vi "Get Next Point.vi"(0 "eye scan point iterator":refnum<class "niHighSpeedSerial Rectangular Eye Scan Point Iterator v1 Host.lvclass">, 11 "error in":errorcluster) -> (4 "eye scan point iterator out":refnum<class "niHighSpeedSerial Rectangular Eye Scan Point Iterator v1 Host.lvclass">, 6 "next point":T1, 15 "error out":errorcluster)   [LabVIEW 2014, in "niHighSpeedSerial Rectangular Eye Scan Point Iterator v1 Host.lvclass"]
doc: "Advances to the next point to be measured and returns its horizontal and vertical offset.\n\n<B>Input Parameters</B>\n\n<B>eye scan point iterator</B> is the incoming wire for the Eye Scan Point Iterator class object\n\n<B>error in</B> describes error conditions that occur before this node runs. This input provides standard 'error in' functionality.\n\n<B>Output Parameters</B>\n\n<B>eye scan point iterator out</B> is the outgoing wire for the Eye Scan Point Iterator class object\n\n<B>next point</B> is the next point to being measuring using Eye Scan\n\n<B>next point.horizontal offset</B> is the horizontal offset of the next point.\n\n<B>next point.vertical offset</B> is the vertical offset of the next point.\n\n<B>error out</B> contains error information. This output provides standard 'error out' functionality."
uses:
  <instrlib>/niHighSpeedSerial/Eye Scan/v1/Host/Impl/Rect Iter/niHighSpeedSerial Rectangular Eye Scan Point Iterator v1 Host.lvclass
  <instrlib>/niHighSpeedSerial/Eye Scan/v1/Host/Common/Public/Point Offsets.ctl
  <instrlib>/niHighSpeedSerial/Eye Scan/v1/Host/Impl/Rect Iter/niHighSpeedSerial Rectangular Eye Scan Point Iterator v1 Host.lvclass/niHighSpeedSerial Rectangular Eye Scan Point Iterator v1 Host.ctl
  <instrlib>/niHighSpeedSerial/Eye Scan/v1/Host/Common/niHighSpeedSerial Eye Scan Common v1 Host.lvlib
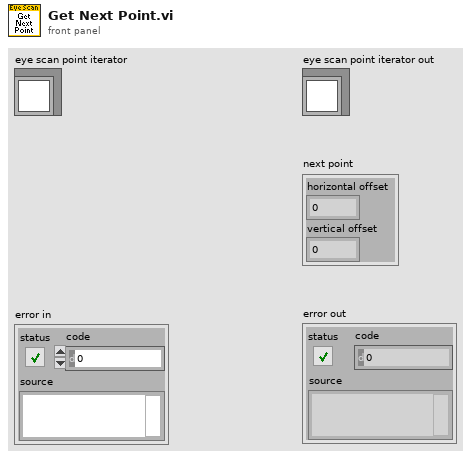
[diagram p1: front panel]
types:
  T1 = typedef "niHighSpeedSerial Eye Scan Common v1 Host.lvlib/Point Offsets.ctl" = cluster{"horizontal offset":i16, "vertical offset":i8}
  T2 = typedef "niHighSpeedSerial Eye Scan Common v1 Host.lvlib/Point.ctl" = cluster{"point offsets":T1, "sample count":u64, "error count":u64, "bit error rate":dbl}
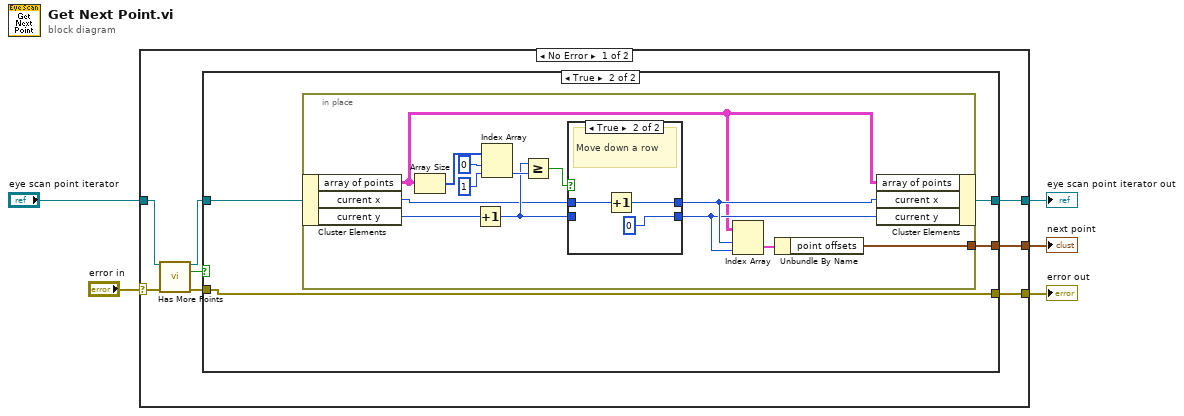
[diagram p0: block diagram]
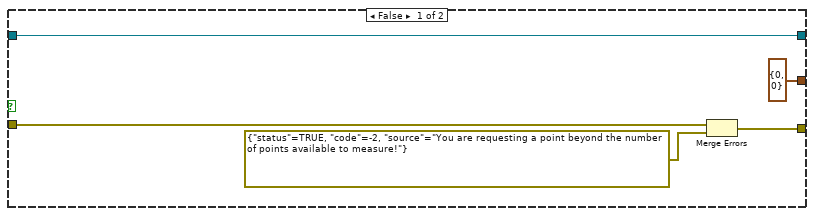
[diagram p2: hidden frame]
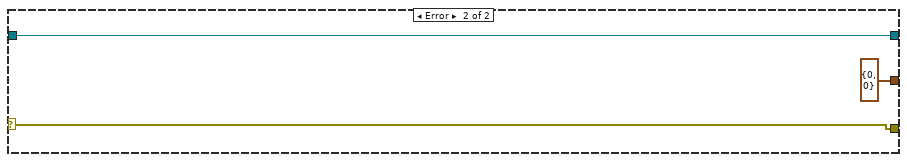
[diagram p4: hidden frame]
diagram:
  n1 = case shown="No Error" "error in" {
    selector: "error in" -> [w8 w43]
    tunnel: [w12 w43] -> w4
    tunnel: [w13 w42] -> w3
    tunnel: "eye scan point iterator" -> [w11 w42]
    tunnel: [w6 T1 {"horizontal offset"=0, "vertical offset"=0} ("Next Point")] -> w1
    frame No Error {
      n2 = call-dynamic "Has More Points.vi"("eye scan point iterator"=w11, "error in"=w8) -> ("eye scan point iterator out"=w10:refnum<class "niHighSpeedSerial Rectangular Eye Scan Point Iterator v1 Host.lvclass">, "has more points?"=w9:bool, "error out"=w7:errorcluster)  [unwired: 11 in]
      n3 = case shown="True" w9 {
        tunnel: [w15 w19] -> w13
        tunnel: [w16 w22] -> w12
        tunnel: w7 -> [w18 w22]
        tunnel: w10 -> [w15 w21]
        tunnel: [T1 {"horizontal offset"=0, "vertical offset"=0} ("Point Offsets") w20] -> w6
        frame False {
          n4 = Merge Errors(w18, errorcluster {"status"=TRUE, "code"=-2, "source"="You are requesting a point beyond the number of points available to measure!"} ("error out")) -> (w16:errorcluster)
        }
        frame True {
          n5 = in-place {
            in-place-border: [w23] -> w20
            n6 = in-place-cluster #1(w21) -> ("array of points"=w24:T2[][], "current x"=w28:i32, "current y"=w27:i32)
            n7 = Array Size(array=w24) -> (size(s)=w30:i32[])
            n8 = Increment(x=w27) -> (x+1=w34:i32)
            n9 = Index Array(array=w30, index #1=0 ("index"), index #2=1 ("index")) -> (element #2=w35:i32)  [unwired: 1 out]
            n10 = Greater Or Equal?(x=w34, y=w35) -> (x >= y?=w33:bool)
            n11 = case shown="True" w33 {
              tunnel: w28 -> [w36 w39]
              tunnel: [w37 0] -> w25
              tunnel: w34 -> [w37 _]
              tunnel: [w36 w38] -> w26
              frame False {
                # "Advance along the row"
              }
              frame True {
                # "Move down a row"
                n12 = Increment(x=w39) -> (x+1=w38:i32)
              }
            }
            n13 = Index Array(array=w24, index (row)=w26, index (col)=w25) -> (element=w29:T2)
            n14 = Unbundle By Name(w29) -> ("point offsets"=w23:T1)
            n15 = in-place-cluster #1("array of points"=w24, "current x"=w26, "current y"=w25) -> (w19:refnum<class "niHighSpeedSerial Rectangular Eye Scan Point Iterator v1 Host.lvclass">)
          }
        }
      }
    }
    frame Error {
    }
  }
  "eye scan point iterator out" <- w3
  "error out" <- w4
  "next point" <- w1
